vi "Handle Message.vi"(8 "error in (no error)":errorcluster, 9 "TcpPayload":T1, 11 "LoggingManager in":refnum<class "LoggingManager.lvclass">) -> (0 "error out":errorcluster, 3 "LoggingManager out":refnum<class "LoggingManager.lvclass">)   [LabVIEW 2020, in "VolatusData.lvlib" / "LoggingManager.lvclass"]
uses:
  LoggingManager.lvclass
  LoggingManager.lvclass/LoggingManager.ctl
  messages/StartLog/StartLog.lvlib
  Volatus/Task/Task.lvclass
  Volatus/Event Level.ctl
  Volatus/Volatus.lvlib
  messages/StopLog/StopLog.lvlib
  C:/dev/lv20CE/relink/lv-volatus/Volatus/Task/Task.lvclass
  C:/Program Files (x86)/National Instruments/LabVIEW 2020/vi.lib/ActorFramework/Actor/Actor.lvclass
  C:/dev/lv20CE/relink/lv-volatus/Volatus/TaskStateHandler/TaskStateHandler.lvclass
  C:/dev/lv20CE/relink/lv-volatus/Volatus/VectoMessageHandler/VectoMessageHandler.lvclass
  C:/dev/lv20CE/relink/lv-volatus/VolatusData/LoggingManager/LoggingManager.lvclass
  C:/dev/lv20CE/relink/lv-volatus/Volatus/API Provider/API Provider.lvclass
  C:/dev/lv20CE/relink/lv-volatus/Volatus/RemoteCommandable/RemoteCommandable.lvclass
  C:/dev/lv20CE/relink/lv-volatus/VolatusData/LoggingHandler/LoggingHandler.lvclass
  lv-vecto/Vecto/proto/TcpPayload/Data.ctl
  lv-vecto/Vecto/proto/TcpPayload/TcpPayload.lvlib
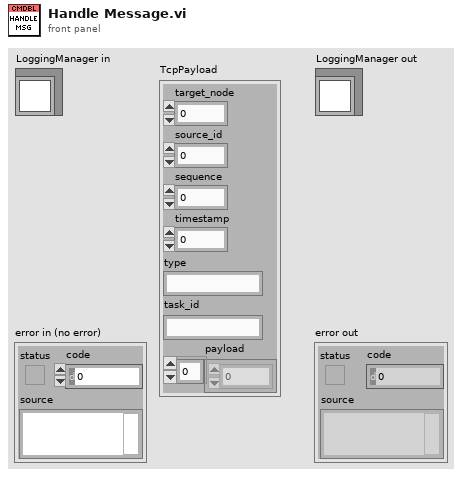
[diagram p1: front panel]
types:
  T1 = typedef "TcpPayload.lvlib/Data.ctl" = cluster{"target_node":u32, "source_id":u32, "sequence":u32, "timestamp":u64, "type":string, "task_id":string, "payload":u8[]}
  T2 = typedef "Volatus.lvlib/Event Level.ctl" = enum16{"Debug", "Info", "Warning", "Error"}
  T3 = typedef "StartLog.lvlib/Data.ctl" = cluster{"series":string, "timestamp":string}
  T4 = typedef "StopLog.lvlib/Data.ctl" = cluster{"reason":string}
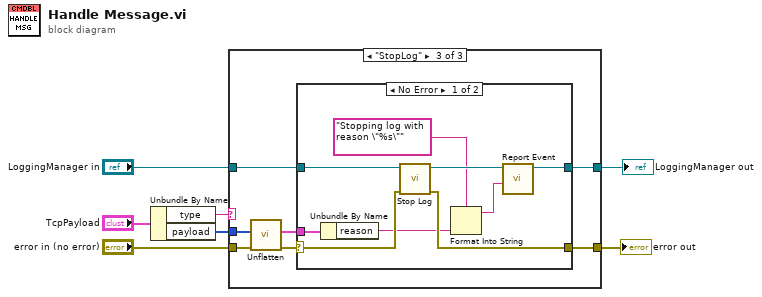
[diagram p0: block diagram]
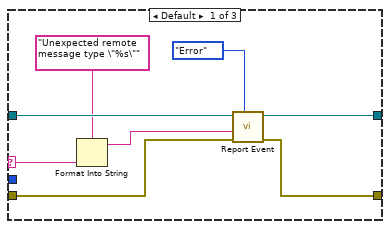
[diagram p2: hidden frame]
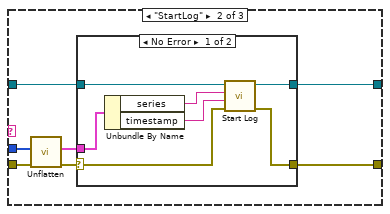
[diagram p3: hidden frame]
diagram:
  n1 = Unbundle By Name("TcpPayload") -> ("type"=w4:string, "payload"=w3:u8[])
  n2 = case shown="\"StopLog\"" w4 {
    selector: w4 -> [w12 _ _]
    tunnel: "error in (no error)" -> [w10 w21 w37]
    tunnel: "LoggingManager in" -> [w15 w18 w34]
    tunnel: w3 -> [_ w22 w38]
    tunnel: [w9 w16 w32] -> w2
    tunnel: [w8 w17 w33] -> w1
    frame Default {
      n3 = Format Into String(format string="Unexpected remote message type \"%s\"", w12) -> (resulting string=w11:string)  [unwired: 2 in, 1 out]
      n4 = call "Report Event.vi"("Level (Info)"=Event_Level."Error", "error in (no error)"=w10, "Message"=w11, "Task in"=w15) -> ("error out"=w9:errorcluster, "Task out"=w8:refnum<class "LoggingManager.lvclass">)  [unwired: 6 in]
    }
    frame "StartLog" {
      n5 = call "Unflatten.vi"("error in"=w21, "Buffer"=w22) -> ("error out"=w19:errorcluster, "Data"=w20:T3)  [unwired: 8 in]
      n6 = case shown="No Error" w19 {
        selector: w19 -> [w25 w30]
        tunnel: w20 -> [w28 _]
        tunnel: w18 -> [w29 w31]
        tunnel: [w24 w31] -> w17
        tunnel: [w23 w30] -> w16
        frame No Error {
          n7 = Unbundle By Name(w28) -> ("series"=w27:string, "timestamp"=w26:string)
          n8 = call-dynamic "Start Log.vi"("error in (no error)"=w25, "Timestamp"=w26, "Series"=w27, "LoggingManager in"=w29) -> ("error out"=w23:errorcluster, "LoggingManager out"=w24:refnum<class "LoggingManager.lvclass">)  [unwired: 6 in]
        }
        frame Error {
        }
      }
    }
    frame "StopLog" {
      n9 = call "Unflatten.vi"("error in"=w37, "Buffer"=w38) -> ("error out"=w35:errorcluster, "Data"=w36:T4)  [unwired: 8 in]
      n10 = case shown="No Error" w35 {
        selector: w35 -> [w45 w48]
        tunnel: w36 -> [w46 _]
        tunnel: w34 -> [w47 w49]
        tunnel: [w40 w49] -> w33
        tunnel: [w43 w48] -> w32
        frame No Error {
          n11 = Unbundle By Name(w46) -> ("reason"=w42:string)
          n12 = call-dynamic "Stop Log.vi"("error in (no error)"=w45, "LoggingManager in"=w47) -> ("error out"=w43:errorcluster, "LoggingManager out"=w44:refnum<class "LoggingManager.lvclass">)  [unwired: 8 in]
          n13 = Format Into String(format string="Stopping log with reason \"%s\"", w42) -> (resulting string=w39:string)  [unwired: 2 in, 1 out]
          n14 = call "Report Event.vi"("Message"=w39, "Task in"=w44) -> ("Task out"=w40:refnum<class "LoggingManager.lvclass">)  [unwired: 8 in, 1 out]
        }
        frame Error {
        }
      }
    }
  }
  "error out" <- w2
  "LoggingManager out" <- w1
